vi "Word Filter Any Letter.vi"() -> ()   [LabVIEW 2015]
uses:
  TypeDef/Letter Statistic.ctl
panel:
  out "size in":i32
  out "size out":i32
  in  "Letters":string
  out "Statistic Letter":T1[](array[typedef])
  out "Dictionary Filter":string[](array[string])
  out "Dictionary":string[](array[string])
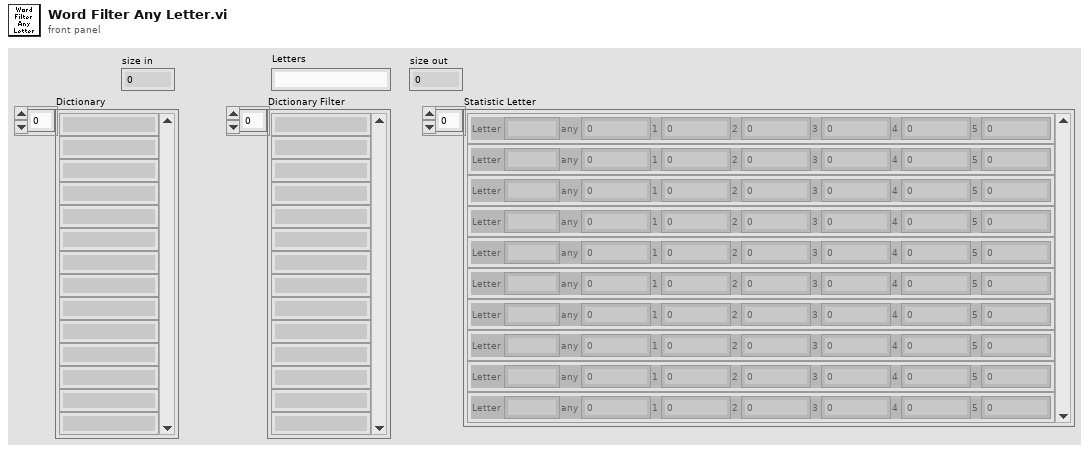
[diagram p1: front panel]
types:
  T1 = typedef "Letter Statistic.ctl" = cluster{"Letter":string, "any":dbl, "1":dbl, "2":dbl, "3":dbl, "4":dbl, "5":dbl}
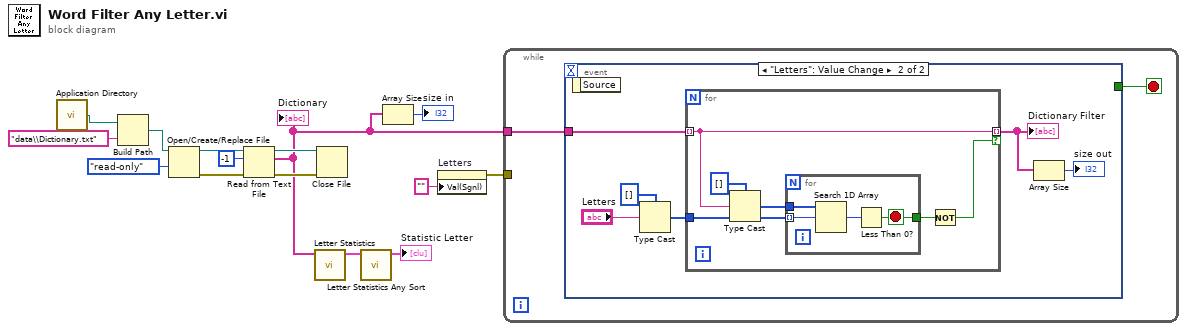
[diagram p0: block diagram]
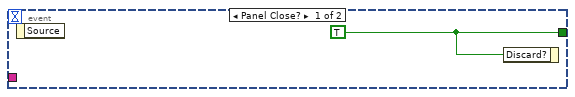
[diagram p2: hidden frame]
diagram:
  n1 = call <vilib>:"Application Directory.vi"() -> ("Application Directory"=w7:path)
  n2 = Build Path(base path=w7, name or relative path="data\\Dictionary.txt") -> (appended path=w9:path)
  n3 = Open/Create/Replace File(file path (use dialog)=w9, access (0:read/write)=enum16{"read/write", "read-only", "write-only"}."read-only") -> (refnum out=w14:refnum<file>, error out=w13:errorcluster)  [unwired: 4 in, 1 out]
  n4 = Read from Text File(file (use dialog)=w14, count=-1, error in=w13) -> (refnum out=w11:refnum<file>, text=w1:string[], error out=w10:errorcluster)  [unwired: 1 in, 1 out]
  "Dictionary" <- w1
  n5 = call "Letter Statistics.vi"("Dictionary"=w1) -> ("Statistic"=w6:T1[])  [unwired: 10 in]
  n6 = Close File(refnum=w11, error in=w10) -> ()  [unwired: 2 out]
  n7 = call "Letter Statistics Any Sort.vi"("Statistic Letter in"=w6) -> ("Statistic Letter out"=→"Statistic Letter":T1[])  [unwired: 10 in]
  n8 = Array Size(array=w1) -> (size(s)=→"size in":i32)
  n9 = property on="Letters" class="Str"("Val(Sgnl)"="" ("Value (Signaling)")) -> (error out=w4:errorcluster)  [unwired: 2 in, 1 out]
  n10 = while {
    tunnel: w1 -> [w16]
    tunnel: w4 -> [_]
    stop <- w17 stop-if-true
    n11 = event shown="[1] \"Letters\": Value Change" {
      selector: _ -> [_ _]
      dyn-events: _ -> [_ _]
      timeout: _ -> [_ _]
      tunnel: [w18 _] -> w17
      tunnel: w16 -> [_ w24]
      event Panel Close? {
        w18 = TRUE
        n12 = event-data() -> ()  [unwired: 1 in, 1 out]
        n13 = event-data("Discard?"=w18) -> ()  [unwired: 1 in, 1 out]
      }
      event "Letters": Value Change {
        n14 = event-data() -> ()  [unwired: 1 in, 1 out]
        n15 = Type Cast(type=u8[] [], x="Letters") -> (*(type *) &x=w21:u8[])
        n16 = for {
          tunnel: w24 -> [w27] mode=indexing
          tunnel: w21 -> [w29]
          tunnel: [w27] -> w20 mode=indexing if=w25
          n17 = Type Cast(type=u8[] [], x=w27) -> (*(type *) &x=w28:u8[])
          n18 = for {
            tunnel: w29 -> [w33] mode=indexing
            tunnel: w28 -> [w34]
            tunnel: [w31] -> w26
            stop <- w31 stop-if-true
            n19 = Search 1D Array(1D array=w34, element=w33) -> (index of element=w32:i32)  [unwired: 1 in]
            n20 = Less Than 0?(x=w32) -> (x < 0?=w31:bool)
          }
          n21 = Not(x=w26) -> (.not. x?=w25:bool)
        }
        "Dictionary Filter" <- w20
        n22 = Array Size(array=w20) -> (size(s)=→"size out":i32)
      }
    }
  }
